vi "Prepare Handlers.vi"(8 "error in (no error)":errorcluster, 11 "DataProcessor in":refnum<class "DataProcessor.lvclass">) -> (0 "error out":errorcluster, 3 "DataProcessor out":refnum<class "DataProcessor.lvclass">)   [LabVIEW 2020, in "VolatusData.lvlib" / "DataProcessor.lvclass"]
uses:
  DataProcessor.lvclass
  DataProcessor.lvclass/DataProcessor.ctl
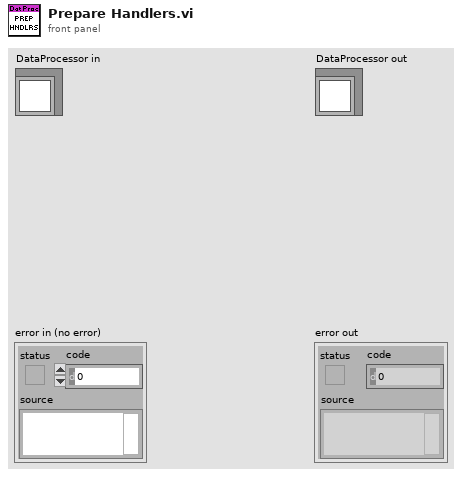
[diagram p1: front panel]
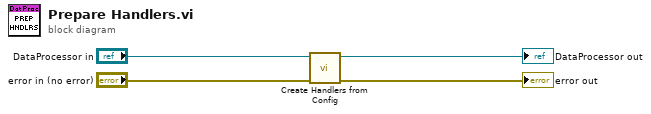
[diagram p0: block diagram]
diagram:
  n1 = call "Create Handlers from Config.vi"("error in (no error)"="error in (no error)", "DataProcessor in"="DataProcessor in") -> ("error out"=→"error out":errorcluster, "DataProcessor out"=→"DataProcessor out":refnum<class "DataProcessor.lvclass">)  [unwired: 8 in]
